vi "校准设置页.vi"() -> ()   [LabVIEW 2016, in "斯坦道CODCr.lvlib"]
uses:
  <vilib>/Analysis/6fits.llb/Curve Fitting Criteria.ctl
  <vilib>/Analysis/NI_AALPro.lvlib
  <vilib>/ptbypt/NI_PtbyPt.lvlib
panel:
  out "校准状态":T1(ring)
  out "模型刷新":bool
  in  "校准按钮":T2(radio)
  in  "校准导入":bool
  in  "辅助计算":bool
  in  "曲线模型":T3={"标液浓度1"=0.0, "测量吸光度1"=0.0, "样品1启用"=FALSE, "标液浓度2"=0.0, "测量吸光度2"=0.0, "样品2启用"=FALSE, "标液浓度3"=0.0, "测量吸光度3"=0.0, "样品3启用"=FALSE, "标液浓度4"=0.0, "测量吸光度4"=0.0, "样品4启用"=FALSE, "标液浓度5"=0.0, "测量吸光度5"=0.0, "样品5启用"=FALSE, "模型"=enum."线性", "精度"=4.0, "XY图"=[], "拟合公式"="", "r^2"=0.0, "标样一校准时间"=timestamp(0 s since 1904-01-01), "标样二校准时间"=timestamp(0 s since 1904-01-01), "标样三校准时间"=timestamp(0 s since 1904-01-01), "标样四校准时间"=timestamp(0 s since 1904-01-01), "标样五校准时间"=timestamp(0 s since 1904-01-01), "二次方程"={"c"=0.0, "x"=0.0, "x^2"=0.0}, "标定时间"=timestamp(0 s since 1904-01-01)} {"标定时间" format="%<%m/%d/%y %H:%M:%S>T"; "标样五校准时间" format="%<%m/%d/%y %H:%M:%S>T"; "标样四校准时间" format="%<%m/%d/%y %H:%M:%S>T"; "标样三校准时间" format="%<%m/%d/%y %H:%M:%S>T"; "标样二校准时间" format="%<%m/%d/%y %H:%M:%S>T"; "标样一校准时间" format="%<%m/%d/%y %H:%M:%S>T"; "r^2" format="%.7f"; "测量吸光度5" format="%#.6f"; "测量吸光度4" format="%#.6f"; "测量吸光度3" format="%#.6f"; "测量吸光度2" format="%#.6f"; "测量吸光度1" format="%#.6f"}
  in  "测量模式":T4(ring)
  in  "参数下拉列表":u16(ring)
  in  "量程下拉列表":enum16{"低量程", "高量程"}(ring)
  # "校准时间"
  # "标液浓度"
  # "吸光值显示"
  # "标液一"
  # "标液二"
  # "标液三"
  # "零点"
  # "跨度"
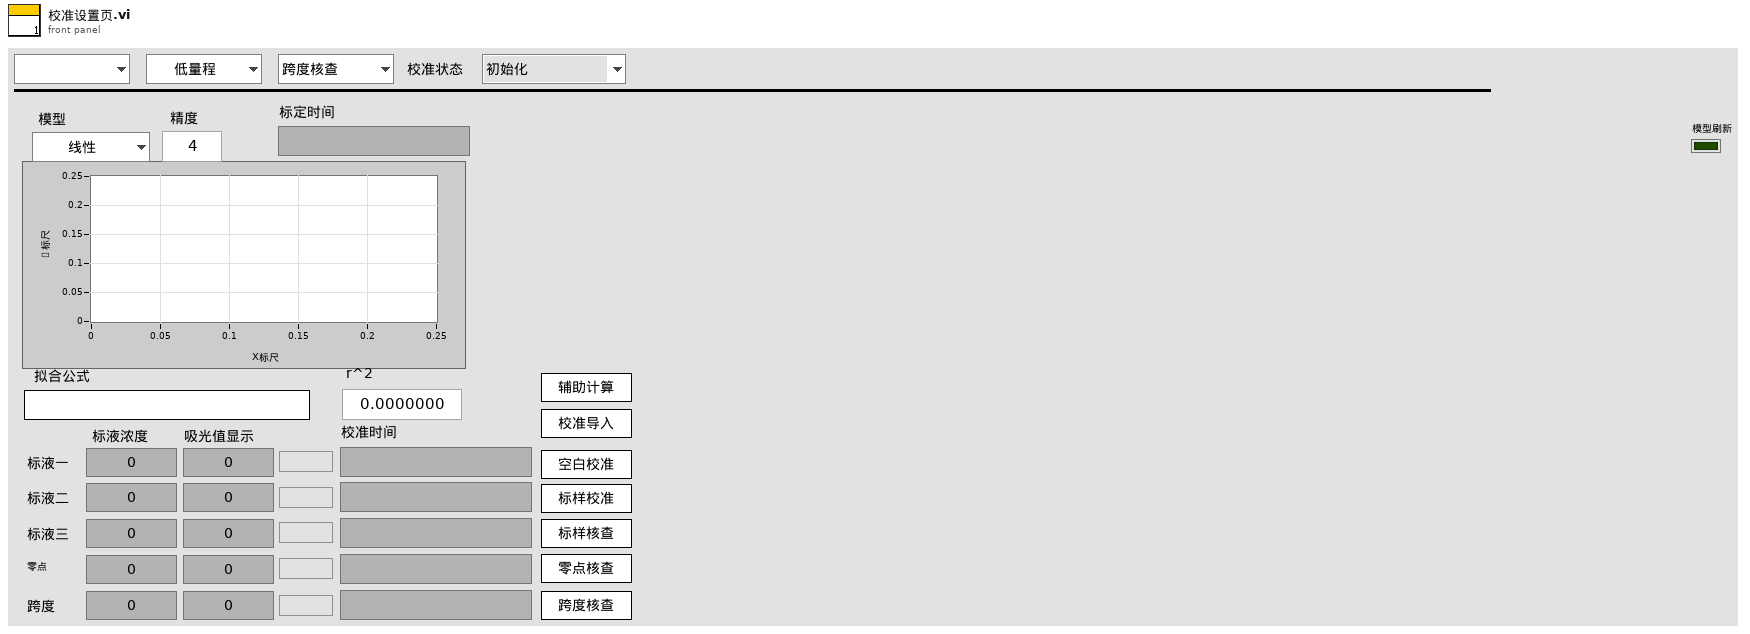
[diagram p1: front panel]
types:
  T1 = enum16{"初始化", "校准启动", "校准运行中", "测试结束", "获取校准数据", "填充校准数据", "流程结束"}
  T2 = enum32{"未选择", "空白校准", "标样校准", "标样核查", "零点核查", "跨度核查"}
  T3 = cluster{"标液浓度1":dbl, "测量吸光度1":dbl, "样品1启用":bool, "标液浓度2":dbl, "测量吸光度2":dbl, "样品2启用":bool, "标液浓度3":dbl, "测量吸光度3":dbl, "样品3启用":bool, "标液浓度4":dbl, "测量吸光度4":dbl, "样品4启用":bool, "标液浓度5":dbl, "测量吸光度5":dbl, "样品5启用":bool, "模型":enum32{"线性", "多项式"}, "精度":dbl, "XY图":cluster{"X Values":dbl[], "Y Values":dbl[]}[], "拟合公式":string, "r^2":dbl, "标样一校准时间":timestamp, "标样二校准时间":timestamp, "标样三校准时间":timestamp, "标样四校准时间":timestamp, "标样五校准时间":timestamp, "二次方程":cluster{"c":dbl, "x":dbl, "x^2":dbl}, "标定时间":timestamp}
  T4 = enum16{"跨度核查", "水样测量", "零点核查", "标样核查", "加标回收", "快捷测试", "空白校准", "标样校准"}
  T5 = typedef "LVStringsAndValuesArrayTypeDef_U16.ctl" = cluster{"String":string, "Value":u16}[]
  T6 = enum8{"Enabled", "Disabled", "Disabled and Grayed Out"}
  T7 = cluster{"标液浓度1":dbl, "测量吸光度1":dbl, "样品1启用":bool, "标液浓度2":dbl, "测量吸光度2":dbl, "样品2启用":bool, "标液浓度3":dbl, "测量吸光度3":dbl, "样品3启用":bool, "标液浓度4":dbl, "测量吸光度4":dbl, "样品4启用":bool, "标液浓度5":dbl, "测量吸光度5":dbl, "样品5启用":bool, "模型":enum32{"线性", "多项式"}, "精度":dbl, "XY图":cluster{"X Values":dbl[], "Y Values":dbl[]}[], "拟合公式":string, "r^2":dbl, "标样一校准时间":timestamp, "标样二校准时间":timestamp, "标样三校准时间":timestamp, "标样四校准时间":timestamp, "标样五校准时间":timestamp, "二次方程":cluster{"c":dbl, "x":dbl, "x^2":dbl}, "标定时间":timestamp}[][]
  T8 = typedef "NI_AALPro.lvlib/Curve Fitting Criteria.ctl" = u16
  T9 = enum32{"Bad", "Idle", "Run top level", "Running"}
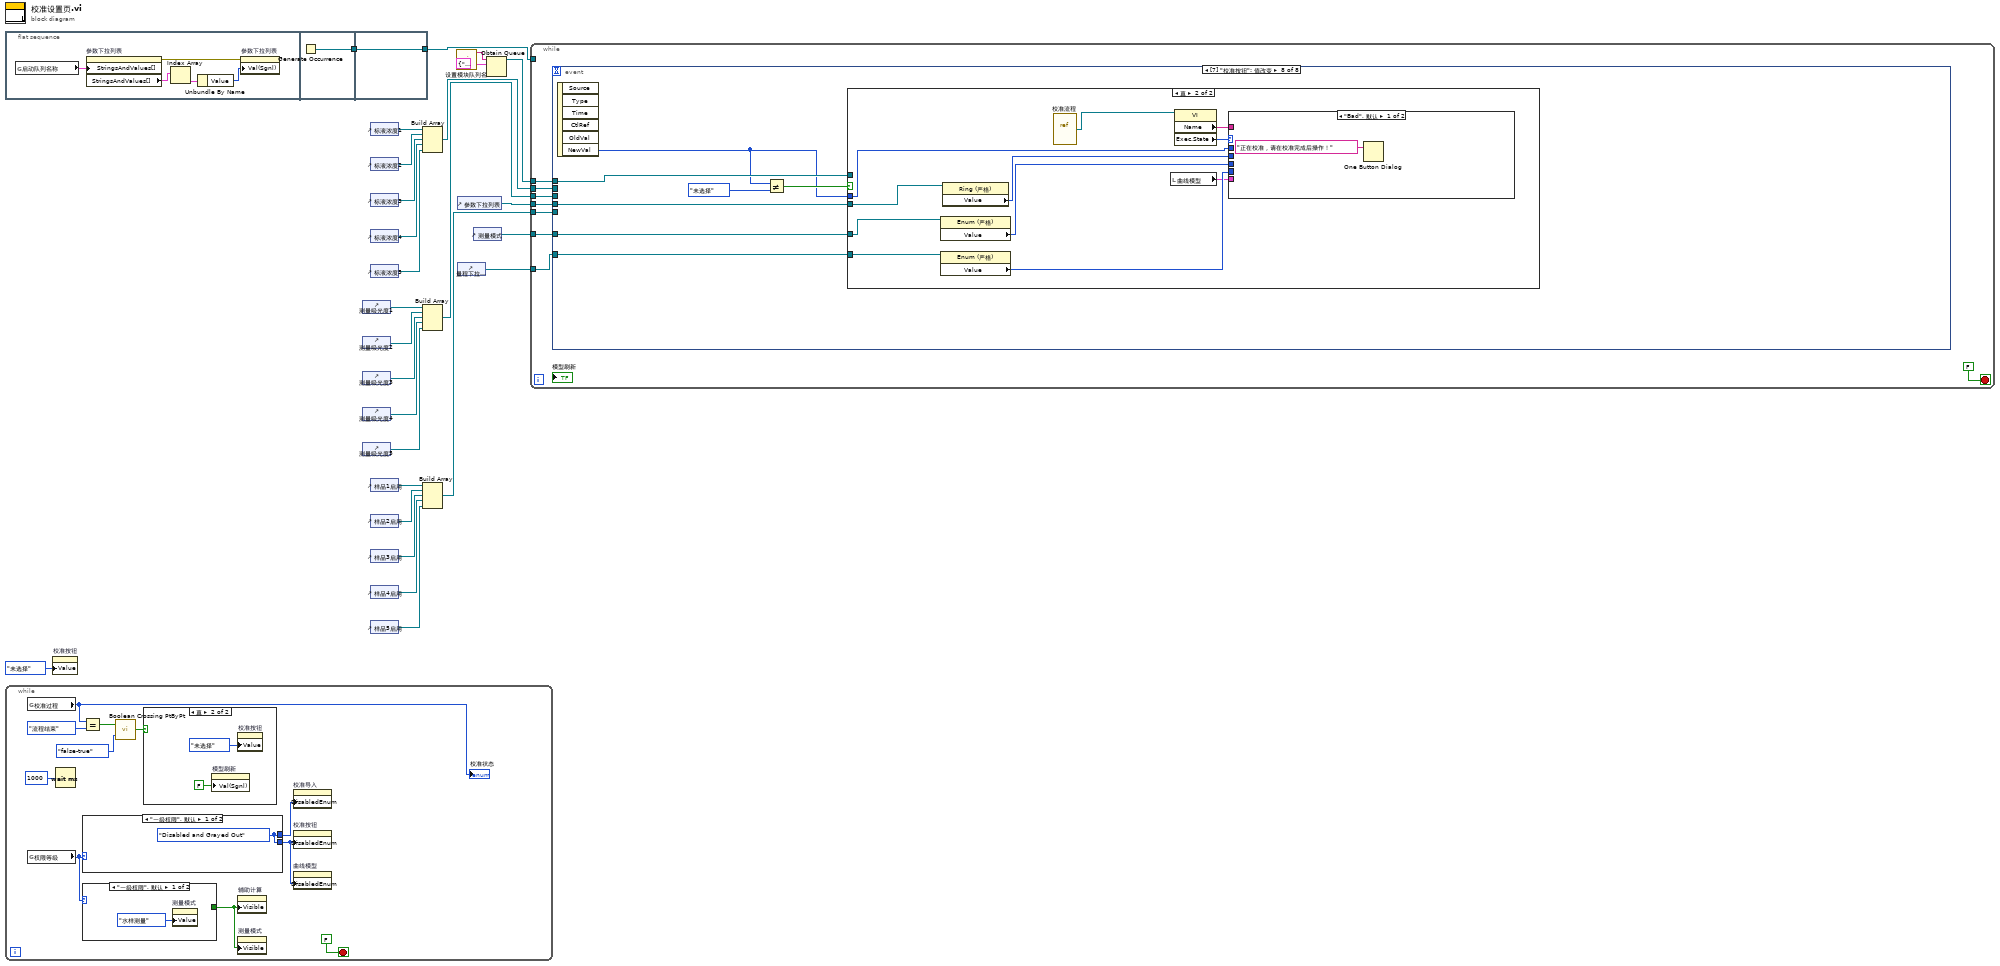
[diagram p0: block diagram]
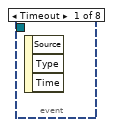
[diagram p2: hidden frame]
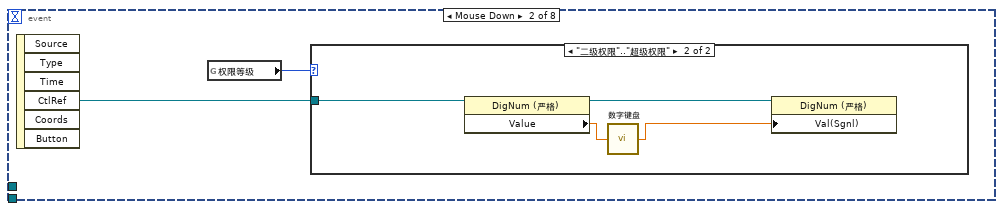
[diagram p3: hidden frame]
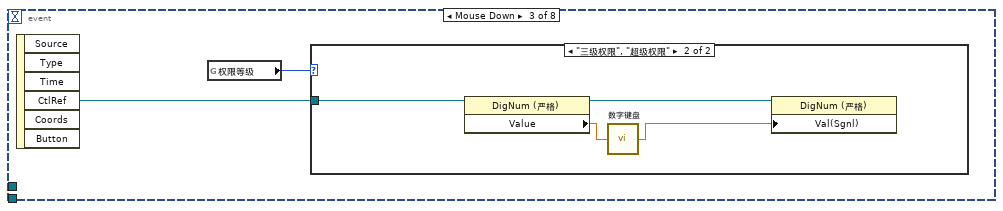
[diagram p5: hidden frame]
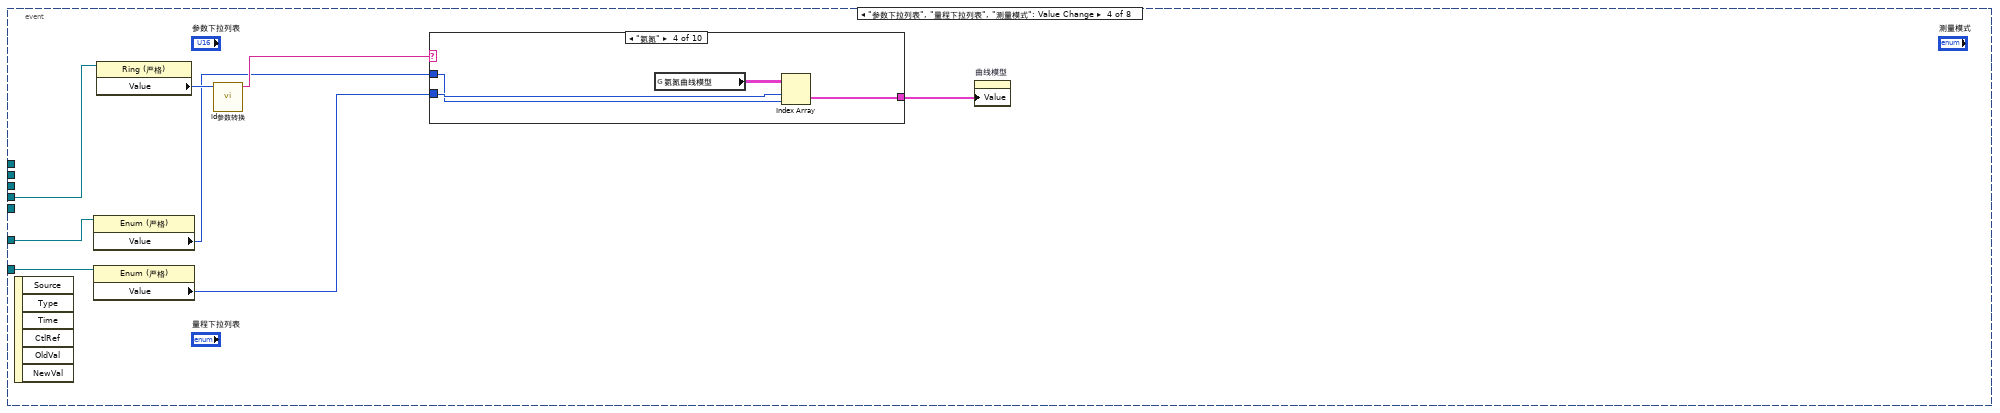
[diagram p7: hidden frame]
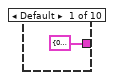
[diagram p8: hidden frame]
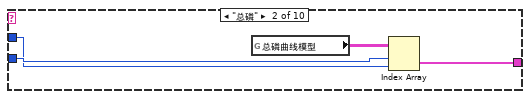
[diagram p9: hidden frame]
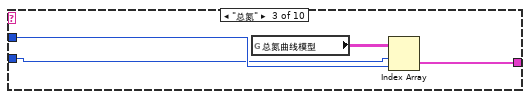
[diagram p10: hidden frame]
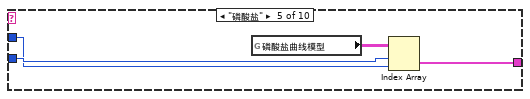
[diagram p11: hidden frame]
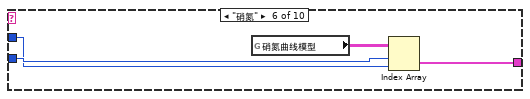
[diagram p12: hidden frame]
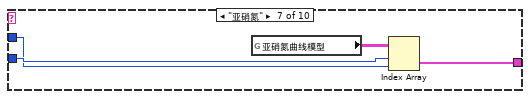
[diagram p13: hidden frame]
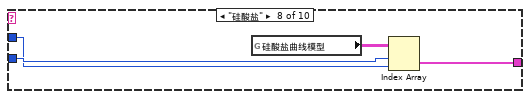
[diagram p14: hidden frame]
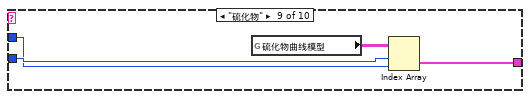
[diagram p15: hidden frame]
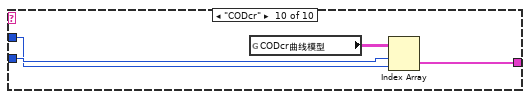
[diagram p16: hidden frame]
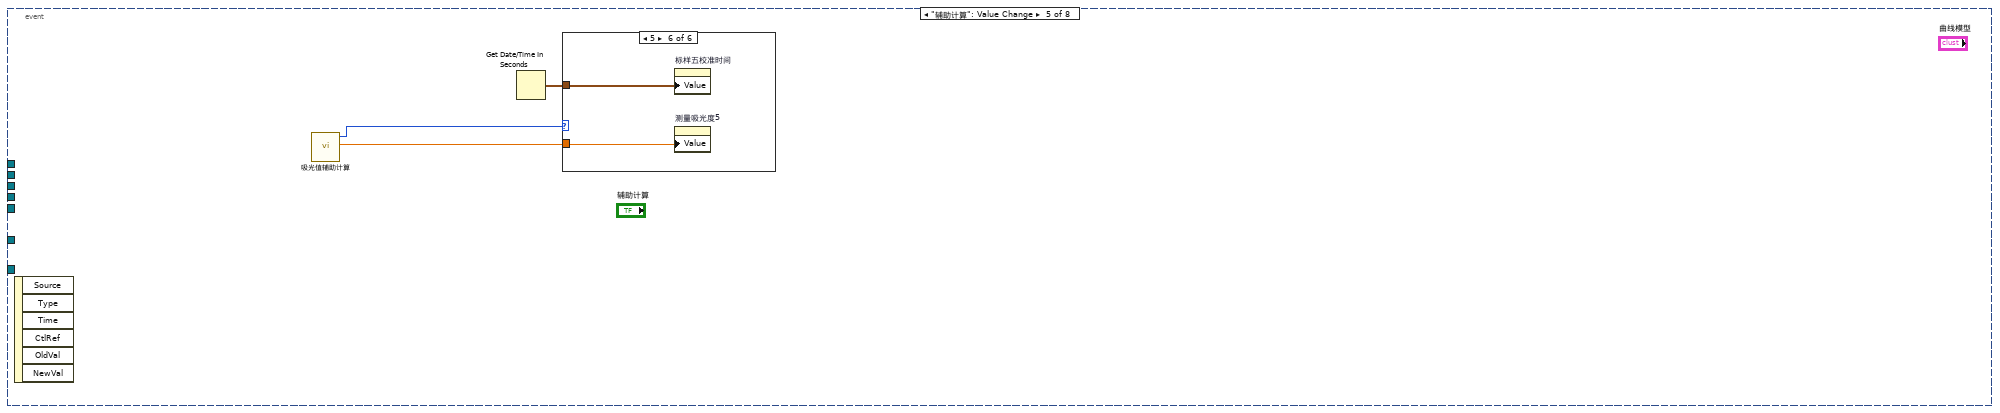
[diagram p17: hidden frame]
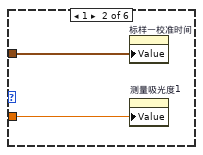
[diagram p19: hidden frame]
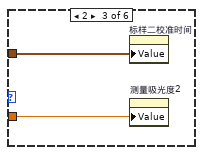
[diagram p20: hidden frame]
diagram:
  n1 = flat-sequence {
    tunnel: [w33] -> w27
    tunnel: [w34] -> w26
    tunnel: w27 -> [w34]
    frame #0 {
      n2 = global read "总磷总氮断电保存全局变量.vi" "启动队列名称"() -> (w28:cluster{"String":string, "Value":u16}[])
      n3 = property on="参数下拉列表" class="Ring (严格)"("StringsAndValues[]"=w28) -> (error out=w31:errorcluster, "StringsAndValues[]"=w29:T5)  [unwired: 2 in, 1 out]
      n4 = Index Array(array=w29) -> (element=w30:cluster{"String":string, "Value":u16})  [unwired: 1 in]
      n5 = Unbundle By Name(w30) -> ("Value"=w32:u16)
      n6 = property on="参数下拉列表" class="Ring (严格)"(error in=w31, "Val(Sgnl)"=w32) -> ()  [unwired: 1 in, 2 out]
    }
    frame #1 {
      n7 = Generate Occurrence() -> (w33:refnum<k4>)
    }
    frame #2 {
    }
  }
  n8 = while {
    stop <- FALSE stop-if-true
    n9 = global read "VAR总磷总氮全局变量.vi" "校准过程"() -> (w35:T1)
    "校准状态" <- w35
    n10 = global read "VAR总磷总氮全局变量.vi" "权限等级"() -> (w42:enum16{"一级权限", "二级权限", "三级权限", "超级权限"})
    n11 = Wait (ms)(milliseconds to wait=u32 1000 ("等待时间（毫秒）")) -> ()  [unwired: 1 out]
    n12 = case shown="\"一级权限\", 默认" w42 {
      tunnel: [w50 w51] -> w40
      tunnel: [w50 w51] -> w43
      frame "一级权限", Default {
        w50 = T6."Disabled and Grayed Out" ("禁用")
      }
      frame "二级权限".."超级权限" {
        w51 = T6."Enabled" ("禁用")
      }
    }
    n13 = case shown="\"一级权限\", 默认" w42 {
      tunnel: [_ TRUE ("可见")] -> w41
      frame "一级权限", Default {
        n14 = property on="测量模式" class="Enum (严格)"("Value"=T4."水样测量" ("测量模式")) -> ()  [unwired: 2 in, 2 out]
      }
      frame "三级权限", "超级权限" {
      }
    }
    n15 = Equal?(x=w35, y=T1."流程结束") -> (x = y?=w38:bool)
    n16 = call <vilib>:"Boolean Crossing PtByPt.vi"("direction"=enum16{"either", "false-true", "true-false"}."false-true", "input"=w38) -> ("crossing"=w36:bool)  [unwired: 1 in]
    n17 = case shown="真" w36 {
      frame False {
      }
      frame True {
        n18 = property on="模型刷新" class="Bool (严格)"("Val(Sgnl)"=FALSE ("值(信号)")) -> ()  [unwired: 2 in, 2 out]
        n19 = property on="校准按钮" class="RadioBtnsControl (严格)"("Value"=T2."未选择" ("校准按钮")) -> ()  [unwired: 2 in, 2 out]
      }
    }
    n20 = property on="辅助计算" class="Bool"("Visible"=w41) -> ()  [unwired: 2 in, 2 out]
    n21 = property on="测量模式" class="Enum (严格)"("Visible"=w41) -> ()  [unwired: 2 in, 2 out]
    n22 = property on="校准导入" class="Bool"("DisabledEnum"=w43) -> ()  [unwired: 2 in, 2 out]
    n23 = property on="校准按钮" class="RadioBtnsControl (严格)"("DisabledEnum"=w40) -> ()  [unwired: 2 in, 2 out]
    n24 = property on="曲线模型" class="Clust (严格)"("DisabledEnum"=w40) -> ()  [unwired: 2 in, 2 out]
  }
  n25 = property on="校准按钮" class="RadioBtnsControl (严格)"("Value"=T2."未选择" ("校准按钮")) -> ()  [unwired: 2 in, 2 out]
  n26 = control-ref of="测量吸光度1"() -> (w14:refnum<vi>)
  n27 = control-ref of="测量吸光度2"() -> (w15:refnum<vi>)
  n28 = control-ref of="测量吸光度3"() -> (w16:refnum<vi>)
  n29 = control-ref of="测量吸光度4"() -> (w17:refnum<vi>)
  n30 = control-ref of="测量吸光度5"() -> (w18:refnum<vi>)
  n31 = control-ref of="标液浓度1"() -> (w12:refnum<vi>)
  n32 = control-ref of="标液浓度2"() -> (w11:refnum<vi>)
  n33 = control-ref of="标液浓度3"() -> (w10:refnum<vi>)
  n34 = control-ref of="标液浓度4"() -> (w9:refnum<vi>)
  n35 = control-ref of="标液浓度5"() -> (w8:refnum<vi>)
  n36 = control-ref of="样品1启用"() -> (w24:refnum<vi>)
  n37 = control-ref of="样品2启用"() -> (w23:refnum<vi>)
  n38 = control-ref of="样品3启用"() -> (w22:refnum<vi>)
  n39 = control-ref of="样品4启用"() -> (w21:refnum<vi>)
  n40 = control-ref of="样品5启用"() -> (w20:refnum<vi>)
  n41 = Build Array(w12, w11, w10, w9, w8) -> (w7:refnum<vi>[])
  n42 = Build Array(w14, w15, w16, w17, w18) -> (w13:refnum<vi>[])
  n43 = Build Array(w24, w23, w22, w21, w20) -> (w19:refnum<vi>[])
  n44 = call "设置模块队列名.vi"() -> ("Msg"=w3:string)  [unwired: 5 in]
  n45 = control-ref of="参数下拉列表"() -> (w25:refnum<vi>)
  n46 = control-ref of="量程下拉列表"() -> (w5:refnum<vi>)
  n47 = control-ref of="测量模式"() -> (w6:refnum<vi>)
  n48 = Obtain Queue(name (unnamed)=w3, element data type=cluster{"命令":string, "data":variant} {"命令"="", "data"=variant}) -> (queue out=w2:refnum<queue>)  [unwired: 3 in, 2 out]
  n49 = while {
    tunnel: w26 -> [_]
    tunnel: w25 -> [w58]
    tunnel: w19 -> [w57]
    tunnel: w13 -> [w56]
    tunnel: w7 -> [w55]
    tunnel: w6 -> [w54]
    tunnel: w5 -> [w53]
    tunnel: w2 -> [w52]
    stop <- FALSE stop-if-true
    n50 = event shown="[7] \"校准按钮\": 值改变" {
      selector: _ -> [_ _ _ _ _ _ _ _]
      dyn-events: _ -> [_ _ _ _ _ _ _ _]
      timeout: _ -> [_ _ _ _ _ _ _ _]
      tunnel: w58 -> [_ _ _ w78 _ w142 w183 w272]
      tunnel: w57 -> [_ _ _ _ _ _ w187 _]
      tunnel: w56 -> [_ _ _ _ _ _ w186 _]
      tunnel: w55 -> [_ _ _ _ _ _ w185 _]
      tunnel: w54 -> [_ _ _ w76 _ w140 w181 w267]
      tunnel: w53 -> [_ _ _ w75 _ w138 w179 w271]
      tunnel: w52 -> [_ _ _ _ _ _ _ w273]
      event Timeout {
        n51 = event-data() -> ()  [unwired: 1 in, 3 out]
      }
      event "曲线模型.标液浓度1", "曲线模型.标液浓度2", "曲线模型.标液浓度3", "曲线模型.标液浓度4", "曲线模型.标液浓度5", "曲线模型.精度": Mouse Down {
        n52 = event-data() -> ("CtlRef"=w61:refnum<vi>)  [unwired: 1 in, 5 out]
        n53 = global read "VAR总磷总氮全局变量.vi" "权限等级"() -> (w60:enum16{"一级权限", "二级权限", "三级权限", "超级权限"})
        n54 = case shown="\"二级权限\"..\"超级权限\"" w60 {
          tunnel: w61 -> [_ w65]
          frame "一级权限", Default {
          }
          frame "二级权限".."超级权限" {
            n55 = property class="DigNum (严格)"(reference=w65) -> (reference out=w63:refnum<vi>, "Value"=w64:dbl)  [unwired: 1 in, 1 out]
            n56 = call "数字键盘.vi"("OldNumber"=w64) -> ("NewNumber"=w62:dbl)
            n57 = property class="DigNum (严格)"(reference=w63, "Val(Sgnl)"=w62) -> ()  [unwired: 1 in, 2 out]
          }
        }
      }
      event "曲线模型.测量吸光度1", "曲线模型.测量吸光度2", "曲线模型.测量吸光度3", "曲线模型.测量吸光度4", "曲线模型.测量吸光度5": Mouse Down {
        n58 = event-data() -> ("CtlRef"=w67:refnum<vi>)  [unwired: 1 in, 5 out]
        n59 = global read "VAR总磷总氮全局变量.vi" "权限等级"() -> (w66:enum16{"一级权限", "二级权限", "三级权限", "超级权限"})
        n60 = case shown="\"三级权限\", \"超级权限\"" w66 {
          tunnel: w67 -> [_ w71]
          frame "一级权限", Default {
          }
          frame "三级权限", "超级权限" {
            n61 = property class="DigNum (严格)"(reference=w71) -> (reference out=w69:refnum<vi>, "Value"=w70:dbl)  [unwired: 1 in, 1 out]
            n62 = call "数字键盘.vi"("OldNumber"=w70) -> ("NewNumber"=w68:dbl)
            n63 = property class="DigNum (严格)"(reference=w69, "Val(Sgnl)"=w68) -> ()  [unwired: 1 in, 2 out]
          }
        }
      }
      event "参数下拉列表", "量程下拉列表", "测量模式": Value Change {
        n64 = event-data() -> ()  [unwired: 1 in, 6 out]
        n65 = property class="Enum (严格)"(reference=w76) -> ("Value"=w73:T4)  [unwired: 1 in, 2 out]
        n66 = property class="Enum (严格)"(reference=w75) -> ("Value"=w74:enum16{"低量程", "高量程"})  [unwired: 1 in, 2 out]
        n67 = property class="Ring (严格)"(reference=w78) -> ("Value"=w79:u16)  [unwired: 1 in, 2 out]
        n68 = call "id参数转换.vi"("id"=w79) -> ("table输出"=w77:string)  [unwired: 9 in, 1 out]
        n69 = case shown="\"氨氮\"" w77 {
          tunnel: w73 -> [_ w83 w88 w90 w94 w98 w102 w106 w110 w114]
          tunnel: w74 -> [_ w84 w87 w91 w95 w99 w103 w107 w111 w115]
          tunnel: [T3 {"标液浓度1"=0.0, "测量吸光度1"=0.0, "样品1启用"=FALSE, "标液浓度2"=0.0, "测量吸光度2"=0.0, "样品2启用"=FALSE, "标液浓度3"=0.0, "测量吸光度3"=0.0, "样品3启用"=FALSE, "标液浓度4"=0.0, "测量吸光度4"=0.0, "样品4启用"=FALSE, "标液浓度5"=0.0, "测量吸光度5"=0.0, "样品5启用"=FALSE, "模型"=enum."线性", "精度"=0.0, "XY图"=[], "拟合公式"="", "r^2"=0.0, "标样一校准时间"=timestamp(0 s since 1904-01-01), "标样二校准时间"=timestamp(0 s since 1904-01-01), "标样三校准时间"=timestamp(0 s since 1904-01-01), "标样四校准时间"=timestamp(0 s since 1904-01-01), "标样五校准时间"=timestamp(0 s since 1904-01-01), "二次方程"={"c"=0.0, "x"=0.0, "x^2"=0.0}, "标定时间"=timestamp(0 s since 1904-01-01)} ("总磷曲线模型") w81 w85 w89 w93 w97 w101 w105 w109 w113] -> w72
          frame Default {
          }
          frame "总磷" {
            n70 = global read "校准数据全局变量.vi" "总磷曲线模型"() -> (w82:T7)
            n71 = Index Array(array=w82, index (row)=w84, index (col)=w83) -> (element=w81:T3)
          }
          frame "总氮" {
            n72 = global read "校准数据全局变量.vi" "总氮曲线模型"() -> (w86:T7)
            n73 = Index Array(array=w86, index (row)=w87, index (col)=w88) -> (element=w85:T3)
          }
          frame "氨氮" {
            n74 = global read "校准数据全局变量.vi" "氨氮曲线模型"() -> (w92:T7)
            n75 = Index Array(array=w92, index (row)=w91, index (col)=w90) -> (element=w89:T3)
          }
          frame "磷酸盐" {
            n76 = global read "校准数据全局变量.vi" "磷酸盐曲线模型"() -> (w96:T7)
            n77 = Index Array(array=w96, index (row)=w95, index (col)=w94) -> (element=w93:T3)
          }
          frame "硝氮" {
            n78 = global read "校准数据全局变量.vi" "硝氮曲线模型"() -> (w100:T7)
            n79 = Index Array(array=w100, index (row)=w99, index (col)=w98) -> (element=w97:T3)
          }
          frame "亚硝氮" {
            n80 = global read "校准数据全局变量.vi" "亚硝氮曲线模型"() -> (w104:T7)
            n81 = Index Array(array=w104, index (row)=w103, index (col)=w102) -> (element=w101:T3)
          }
          frame "硅酸盐" {
            n82 = global read "校准数据全局变量.vi" "硅酸盐曲线模型"() -> (w108:T7)
            n83 = Index Array(array=w108, index (row)=w107, index (col)=w106) -> (element=w105:T3)
          }
          frame "硫化物" {
            n84 = global read "校准数据全局变量.vi" "硫化物曲线模型"() -> (w112:T7)
            n85 = Index Array(array=w112, index (row)=w111, index (col)=w110) -> (element=w109:T3)
          }
          frame "CODcr" {
            n86 = global read "校准数据全局变量.vi" "CODcr曲线模型"() -> (w116:T7)
            n87 = Index Array(array=w116, index (row)=w115, index (col)=w114) -> (element=w113:T3)
          }
        }
        n88 = property on="曲线模型" class="Clust (严格)"("Value"=w72) -> ()  [unwired: 2 in, 2 out]
      }
      event "辅助计算": Value Change {
        n89 = event-data() -> ()  [unwired: 1 in, 6 out]
        n90 = call "吸光值辅助计算.vi"() -> ("X"=w118:dbl, "吸光值导出"=w119:u16)  [unwired: 10 in]
        n91 = Get Date/Time In Seconds() -> (seconds since 1Jan1904=w117:timestamp)
        n92 = case shown="5" w119 {
          tunnel: w118 -> [_ w121 w123 w125 w127 w129]
          tunnel: w117 -> [_ w120 w122 w124 w126 w128]
          frame 0, Default {
          }
          frame 1 {
            n93 = property on="标样一校准时间" class="AbsTime (严格)"("Value"=w120) -> ()  [unwired: 2 in, 2 out]
            n94 = property on="测量吸光度1" class="DigNum (严格)"("Value"=w121) -> ()  [unwired: 2 in, 2 out]
          }
          frame 2 {
            n95 = property on="标样二校准时间" class="AbsTime (严格)"("Value"=w122) -> ()  [unwired: 2 in, 2 out]
            n96 = property on="测量吸光度2" class="DigNum (严格)"("Value"=w123) -> ()  [unwired: 2 in, 2 out]
          }
          frame 3 {
            n97 = property on="标样三校准时间" class="AbsTime (严格)"("Value"=w124) -> ()  [unwired: 2 in, 2 out]
            n98 = property on="测量吸光度3" class="DigNum (严格)"("Value"=w125) -> ()  [unwired: 2 in, 2 out]
          }
          frame 4 {
            n99 = property on="标样四校准时间" class="AbsTime (严格)"("Value"=w126) -> ()  [unwired: 2 in, 2 out]
            n100 = property on="测量吸光度4" class="DigNum (严格)"("Value"=w127) -> ()  [unwired: 2 in, 2 out]
          }
          frame 5 {
            n101 = property on="标样五校准时间" class="AbsTime (严格)"("Value"=w128) -> ()  [unwired: 2 in, 2 out]
            n102 = property on="测量吸光度5" class="DigNum (严格)"("Value"=w129) -> ()  [unwired: 2 in, 2 out]
          }
        }
      }
      event "校准导入": Value Change {
        n103 = event-data() -> ()  [unwired: 1 in, 6 out]
        n104 = property class="Enum (严格)"(reference=w140) -> ("Value"=w139:T4)  [unwired: 1 in, 2 out]
        n105 = property class="Enum (严格)"(reference=w138) -> ("Value"=w137:enum16{"低量程", "高量程"})  [unwired: 1 in, 2 out]
        n106 = property class="Ring (严格)"(reference=w142) -> ("Value"=w141:u16)  [unwired: 1 in, 2 out]
        n107 = property on="二次方程" class="Clust (严格)"() -> ("Value"=w131:cluster{"c":dbl, "x":dbl, "x^2":dbl})  [unwired: 2 in, 2 out]
        n108 = Unbundle By Name(w131) -> ("x^2"=w133:dbl, "x"=w134:dbl, "c"=w135:dbl)
        n109 = Bundle By Name(cluster=cluster{"X^2":dbl, "X":dbl, "b":dbl} {"X^2"=0.0, "X"=0.0, "b"=0.0} ("公式"), "X^2"=w133, "X"=w134, "b"=w135) -> (w130:cluster{"X^2":dbl, "X":dbl, "b":dbl})
        n110 = global read "VAR总磷总氮全局变量.vi" "权限等级"() -> (w136:enum16{"一级权限", "二级权限", "三级权限", "超级权限"})
        n111 = case shown="\"一级权限\", 默认" w136 {
          tunnel: w141 -> [w151 w178]
          tunnel: w139 -> [w150 w177]
          tunnel: w137 -> [w149 w176]
          tunnel: w130 -> [w143 _]
          frame "一级权限", Default {
            n112 = Cluster To Array(cluster=w143) -> (array=w148:dbl[])
            n113 = Add Array Elements(numeric array=w148) -> (sum=w147:dbl)
            n114 = Equal To 0?(x=w147) -> (x = 0?=w145:bool)
            n115 = Not A Number/Path/Refnum?(number/path/refnum=w147) -> (NaN/Path/Refnum?=w146:bool)
            n116 = Or(x=w145, y=w146) -> (x .or. y?=w144:bool)
            n117 = case shown="假" w144 {
              tunnel: w151 -> [w157 _]
              tunnel: w150 -> [w156 _]
              tunnel: w149 -> [w155 _]
              tunnel: w143 -> [w152 _]
              frame False {
                n118 = Two Button Dialog(message="请再一次确认是否导入" ("消息")) -> (T button?=w153:bool)  [unwired: 2 in]
                n119 = case shown="真" w153 {
                  tunnel: w157 -> [_ w165]
                  tunnel: w156 -> [_ w164]
                  tunnel: w155 -> [_ w163]
                  tunnel: w152 -> [_ w158]
                  frame False {
                  }
                  frame True {
                    n120 = for {
                      N: 8 -> [_]
                      tunnel: w165 -> [w171]
                      tunnel: w164 -> [_]
                      tunnel: w163 -> [w170]
                      shift-right: [w169] -> w161
                      shift-left: errorcluster {"status"=FALSE, "code"=0, "source"=""} ("error out") -> [w166]
                      tunnel: w158 -> [w167]
                      i -> [w168]
                      n121 = call "总磷总氮公式写入.vi"("公式"=w167, "error in (no error)"=w166, "量程"=w170, "测量模式"=w168, "测量参数"=w171) -> ("error out"=w169:errorcluster)  [unwired: 6 in]
                    }
                    n122 = case shown="无错误" w161 {
                      tunnel: ["写入成功" "写入失败"] -> w162
                      frame No Error {
                        n123 = Get Date/Time In Seconds() -> (seconds since 1Jan1904=w172:timestamp)
                        n124 = property on="标定时间" class="AbsTime (严格)"("Value"=w172) -> ()  [unwired: 2 in, 2 out]
                      }
                      frame Error {
                      }
                    }
                    n125 = One Button Dialog(message=w162) -> ()  [unwired: 1 in, 1 out]
                  }
                }
              }
              frame True {
                n126 = One Button Dialog(message="校准数据异常，请重新校准！" ("消息")) -> ()  [unwired: 1 in, 1 out]
              }
            }
          }
          frame "三级权限", "超级权限" {
            n127 = call "公式复合写入.vi"("量程下拉列表"=w176, "测量模式"=w177, "参数下拉列表"=w178) -> ()  [unwired: 9 in]
          }
        }
      }
      event "曲线模型", "模型刷新": Value Change {
        n128 = event-data() -> ()  [unwired: 1 in, 6 out]
        n129 = flat-sequence {
          tunnel: w187 -> [w207]
          tunnel: w186 -> [w205]
          tunnel: w185 -> [w203]
          tunnel: [w190] -> w184
          tunnel: w183 -> [w190]
          tunnel: [w189] -> w182
          tunnel: w181 -> [w189]
          tunnel: [w188] -> w180
          tunnel: w179 -> [w188]
          tunnel: w184 -> [w221]
          tunnel: w182 -> [w217]
          tunnel: w180 -> [w216]
          frame #0 {
            w199 = T8 0 items=["最小二乘", "最小绝对残差", "Bisquare"] ("method")
            n130 = for {
              tunnel: w207 -> [w213] mode=indexing
              tunnel: [w212] -> w206 mode=indexing
              tunnel: w205 -> [w211] mode=indexing
              tunnel: [w210] -> w204 mode=indexing
              tunnel: w203 -> [w209] mode=indexing
              tunnel: [w208] -> w202 mode=indexing
              n131 = property class="DigNum (严格)"(reference=w209) -> ("Value"=w208:dbl)  [unwired: 1 in, 2 out]
              n132 = property class="DigNum (严格)"(reference=w211) -> ("Value"=w210:dbl)  [unwired: 1 in, 2 out]
              n133 = property class="Bool (严格)"(reference=w213) -> ("Value"=w212:bool)  [unwired: 1 in, 2 out]
            }
            n134 = property on="模型" class="Enum (严格)"() -> ("Value"=w201:enum32{"线性", "多项式"})  [unwired: 2 in, 2 out]
            n135 = property on="精度" class="DigNum (严格)"() -> ("Value"=w200:dbl)  [unwired: 2 in, 2 out]
            n136 = call "线性公式.vi"("精度"=w200, "模型"=w201, "method"=w199, "启用"=w206, "监测浓度"=w204, "标液浓度"=w202) -> ("Polynomial Coefficients 2"=w195:dbl[], "XY图"=w196:cluster{"X Values":dbl[], "Y Values":dbl[]}[], "r^2"=w197:dbl, "拟合方程"=w198:string)  [unwired: 2 in]
            n137 = property on="拟合公式" class="Str"("Value"=w198) -> ()  [unwired: 2 in, 2 out]
            n138 = property on="r^2" class="DigNum (严格)"("Value"=w197) -> ()  [unwired: 2 in, 2 out]
            n139 = property on="XY图" class="XYGraph (严格)"("Value"=w196) -> ()  [unwired: 2 in, 2 out]
            n140 = Index Array(array=w195) -> (element #1=w194:dbl, element #2=w193:dbl, element #3=w192:dbl)  [unwired: 3 in]
            n141 = Bundle("slope"=w194, "slope"=w193, "slope"=w192) -> (w191:cluster{"slope":dbl, "slope":dbl, "slope":dbl})  [unwired: 1 in]
            n142 = property on="二次方程" class="Clust (严格)"("Value"=w191) -> ()  [unwired: 2 in, 2 out]
          }
          frame #1 {
            n143 = property class="Enum (严格)"(reference=w217) -> ("Value"=w214:T4)  [unwired: 1 in, 2 out]
            n144 = property class="Enum (严格)"(reference=w216) -> ("Value"=w215:enum16{"低量程", "高量程"})  [unwired: 1 in, 2 out]
            n145 = property class="Ring (严格)"(reference=w221) -> ("Value"=w220:u16)  [unwired: 1 in, 2 out]
            n146 = call "id参数转换.vi"("id"=w220) -> ("table输出"=w219:string)  [unwired: 9 in, 1 out]
            n147 = property on="曲线模型" class="Clust (严格)"() -> ("Value"=w218:T3)  [unwired: 2 in, 2 out]
            n148 = case shown="\"总磷\"" w219 {
              tunnel: w218 -> [_ w226 w231 w233 w237 w242 w247 w252 w257 w263]
              tunnel: w215 -> [_ w224 w230 w234 w238 w243 w248 w253 w258 w264]
              tunnel: w214 -> [_ w225 w229 w235 w239 w244 w249 w254 w259 w265]
              frame Default {
              }
              frame "总磷" {
                n149 = global read "校准数据全局变量.vi" "总磷曲线模型"() -> (w222:T7)
                n150 = Replace Array Subset(array=w222, new element=w226, index (row)=w225, index (col)=w224) -> (w223:T7)
                n151 = global write "校准数据全局变量.vi" "总磷曲线模型"(w223) -> ()
              }
              frame "总氮" {
                n152 = global read "校准数据全局变量.vi" "总氮曲线模型"() -> (w228:T7)
                n153 = Replace Array Subset(array=w228, new element=w231, index (row)=w229, index (col)=w230) -> (w227:T7)
                n154 = global write "校准数据全局变量.vi" "总氮曲线模型"(w227) -> ()
              }
              frame "氨氮" {
                n155 = global read "校准数据全局变量.vi" "氨氮曲线模型"() -> (w236:T7)
                n156 = Replace Array Subset(array=w236, new element=w233, index (row)=w235, index (col)=w234) -> (w232:T7)
                n157 = global write "校准数据全局变量.vi" "氨氮曲线模型"(w232) -> ()
              }
              frame "磷酸盐" {
                n158 = global read "校准数据全局变量.vi" "磷酸盐曲线模型"() -> (w241:T7)
                n159 = Replace Array Subset(array=w241, new element=w237, index (row)=w239, index (col)=w238) -> (w240:T7)
                n160 = global write "校准数据全局变量.vi" "磷酸盐曲线模型"(w240) -> ()
              }
              frame "硝氮" {
                n161 = global read "校准数据全局变量.vi" "硝氮曲线模型"() -> (w246:T7)
                n162 = Replace Array Subset(array=w246, new element=w242, index (row)=w244, index (col)=w243) -> (w245:T7)
                n163 = global write "校准数据全局变量.vi" "硝氮曲线模型"(w245) -> ()
              }
              frame "亚硝氮" {
                n164 = global read "校准数据全局变量.vi" "亚硝氮曲线模型"() -> (w251:T7)
                n165 = Replace Array Subset(array=w251, new element=w247, index (row)=w249, index (col)=w248) -> (w250:T7)
                n166 = global write "校准数据全局变量.vi" "亚硝氮曲线模型"(w250) -> ()
              }
              frame "硅酸盐" {
                n167 = global read "校准数据全局变量.vi" "硅酸盐曲线模型"() -> (w256:T7)
                n168 = Replace Array Subset(array=w256, new element=w252, index (row)=w254, index (col)=w253) -> (w255:T7)
                n169 = global write "校准数据全局变量.vi" "硅酸盐曲线模型"(w255) -> ()
              }
              frame "硫化物" {
                n170 = global read "校准数据全局变量.vi" "硫化物曲线模型"() -> (w261:T7)
                n171 = Replace Array Subset(array=w261, new element=w257, index (row)=w259, index (col)=w258) -> (w260:T7)
                n172 = global write "校准数据全局变量.vi" "硫化物曲线模型"(w260) -> ()
              }
              frame "CODcr" {
                n173 = global read "校准数据全局变量.vi" "CODcr曲线模型"() -> (w266:T7)
                n174 = Replace Array Subset(array=w266, new element=w263, index (row)=w265, index (col)=w264) -> (w262:T7)
                n175 = global write "校准数据全局变量.vi" "CODcr曲线模型"(w262) -> ()
              }
            }
          }
          frame #2 {
            n176 = call "校准数据写入配置文件.vi"() -> ()  [unwired: 11 in, 1 out]
          }
        }
      }
      event "校准按钮": Value Change {
        n177 = event-data() -> ("NewVal"=w268:T2)  [unwired: 1 in, 5 out]
        n178 = Not Equal?(x=w268, y=T2."未选择") -> (x != y?=w269:bool)
        n179 = case shown="真" w269 {
          tunnel: w273 -> [_ _]
          tunnel: w272 -> [_ w284]
          tunnel: w271 -> [_ w283]
          tunnel: w268 -> [_ w278]
          tunnel: w267 -> [_ w282]
          frame False {
          }
          frame True {
            n180 = property class="Enum (严格)"(reference=w282) -> ("Value"=w276:T4)  [unwired: 1 in, 2 out]
            n181 = property class="Enum (严格)"(reference=w283) -> ("Value"=w275:enum16{"低量程", "高量程"})  [unwired: 1 in, 2 out]
            n182 = property class="Ring (严格)"(reference=w284) -> ("Value"=w277:u16)  [unwired: 1 in, 2 out]
            n183 = vi-ref "校准流程.vi"() -> (w279:refnum<vi>)
            n184 = local read "曲线模型"() -> (w274:T3)
            n185 = property class="VI"(reference=w279) -> ("Name"=w280:string, "Exec.State"=w281:T9)  [unwired: 1 in, 2 out]
            n186 = case shown="\"Bad\", 默认" w281 {
              tunnel: w280 -> [_ w297]
              tunnel: w278 -> [_ w290]
              tunnel: w277 -> [_ w289]
              tunnel: w276 -> [_ w288]
              tunnel: w275 -> [_ w287]
              tunnel: w274 -> [_ w286]
              frame "Bad", Default {
                n187 = One Button Dialog(message="正在校准，请在校准完成后操作！" ("消息")) -> ()  [unwired: 1 in, 1 out]
              }
              frame "Idle" {
                n188 = Open VI Reference(type specifier VI Refnum (for type only)=refnum<vi> refnum, vi path=w297, options=128 ("选项")) -> (vi reference=w295:refnum<vi>, error out=w294:errorcluster)  [unwired: 3 in]
                n189 = call-by-ref "开始异步调用"(reference=w295, error in=w294, "校准模式"=w290, "参数下拉列表"=w289, "测量模式"=w288, "量程下拉列表"=w287, "曲线模型"=w286) -> (reference out=w292:refnum<vi>, error out=w293:errorcluster)  [unwired: 11 in]
                n190 = Close Reference(reference=w292, error in (no error)=w293) -> ()  [unwired: 1 out]
              }
            }
          }
        }
      }
    }
  }
